vi "PH_GUI.set I32 GUI object.vi"(0 "Caption.Text [Empty]":string, 1 "Visible (true)":bool=TRUE, 2 "I32 GUI Ref":refnum<vi>, 3 "value":i32, 4 "blinking (false)":bool, 5 "error in (no error)":errorcluster, 7 "Tip Strip [Empty]":string, 9 "Disabled (Enabled)":T1(ring)) -> (19 "error out":errorcluster)   [LabVIEW 2014, in "PH_Common.lvlib"]
doc: "Sets value and more for the referenced GUI object."
uses:
  PH_Common.lvlib
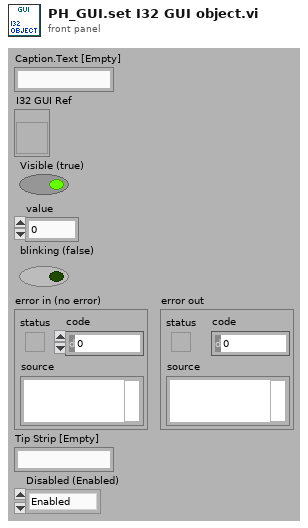
[diagram p1: front panel]
types:
  T1 = enum8{"Enabled", "Disabled", "Disabled and Grayed Out"}
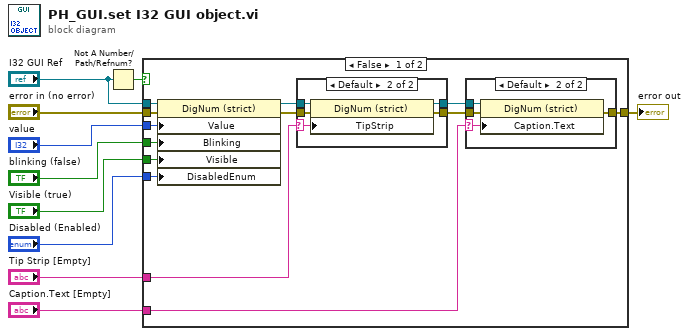
[diagram p0: block diagram]
diagram:
  n1 = Not A Number/Path/Refnum?(number/path/refnum="I32 GUI Ref") -> (NaN/Path/Refnum?=w7:bool)
  n2 = case shown="False" w7 {
    tunnel: "I32 GUI Ref" -> [w22 _]
    tunnel: "error in (no error)" -> [w23 w36]
    tunnel: [w15 w36] -> w9
    tunnel: "value" -> [w21 _]
    tunnel: "blinking (false)" -> [w20 _]
    tunnel: "Visible (true)" -> [w19 _]
    tunnel: "Disabled (Enabled)" -> [w18 _]
    tunnel: "Tip Strip [Empty]" -> [w12 _]
    tunnel: "Caption.Text [Empty]" -> [w11 _]
    frame False {
      n3 = property class="DigNum (strict)"(reference=w22, error in=w23, "Value"=w21, "Blinking"=w20, "Visible"=w19, "DisabledEnum"=w18) -> (reference out=w14:refnum<vi>, error out=w16:errorcluster)
      n4 = case shown="Default" w12 {
        selector: w12 -> [_ w31]
        tunnel: [w29 w35] -> w17
        tunnel: w16 -> [w29 w34]
        tunnel: w14 -> [w30 w33]
        tunnel: [w30 w32] -> w13
        frame "", "N/A" {
        }
        frame Default {
          n5 = property class="DigNum (strict)"(reference=w33, error in=w34, "TipStrip"=w31) -> (reference out=w32:refnum<vi>, error out=w35:errorcluster)
        }
      }
      n6 = case shown="Default" w11 {
        selector: w11 -> [_ w25]
        tunnel: w17 -> [w24 w28]
        tunnel: [w24 w27] -> w15
        tunnel: w13 -> [_ w26]
        frame "", "N/A" {
        }
        frame Default {
          n7 = property class="DigNum (strict)"(reference=w26, error in=w28, "Caption.Text"=w25) -> (error out=w27:errorcluster)  [unwired: 1 out]
        }
      }
    }
    frame True {
    }
  }
  "error out" <- w9
